vi "Error Query.vi"(0 "VISA resource name":refnum<visa-resource-name>, 11 "error in (no error)":errorcluster) -> (4 "VISA resource name out":refnum<visa-resource-name>, 8 "Error":i32, 10 "Error Message":string, 15 "error out":errorcluster)   [LabVIEW 2020, in "Stanford Research PS300 Series.lvlib"]
doc: "This instrument does not support an error query and will return a warning if this VI is called."
uses:
  Stanford Research PS300 Series.lvlib
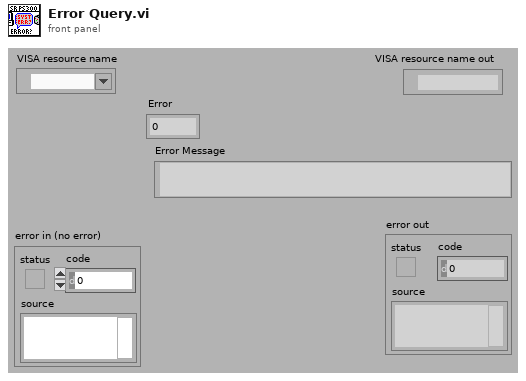
[diagram p1: front panel]
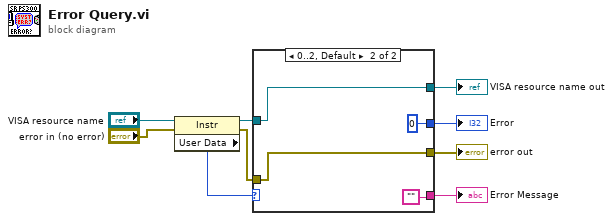
[diagram p0: block diagram]
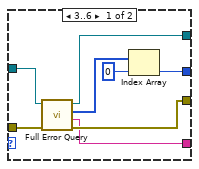
[diagram p2: hidden frame]
diagram:
  n1 = property class="Instr"(reference="VISA resource name", error in="error in (no error)") -> (reference out=w3:refnum<visa-resource-name>, error out=w5:errorcluster, "User Data"=w4:u32)
  n2 = case shown="0..2, Default" w4 {
    tunnel: [w10 0] -> w1
    tunnel: w5 -> [w15 w19]
    tunnel: [w14 w19] -> w9
    tunnel: [w13 ""] -> w8
    tunnel: w3 -> [w17 w21]
    tunnel: [w16 w21] -> w2
    frame 3..6 {
      n3 = call "Full Error Query.vi"("error in (no error)"=w15, "VISA resource name"=w17) -> ("error out"=w14:errorcluster, "Error Message"=w13:string, "Error Code"=w12:i32[], "VISA resource name out"=w16:refnum<visa-resource-name>)  [unwired: 6 in]
      n4 = Index Array(array=w12, index=0) -> (element=w10:i32)
    }
    frame 0..2, Default {
    }
  }
  "Error Message" <- w8
  "Error" <- w1
  "VISA resource name out" <- w2
  "error out" <- w9
